vi "Query-ControlSignal.vi"(8 "error in (no error)":errorcluster, 10 "Output channel":T1, 11 "VISA resource name":refnum<visa-resource-name>) -> (0 "error out":errorcluster, 2 "Recalled Control signal / V":dbl, 3 "VISA resource name out":refnum<visa-resource-name>)   [LabVIEW 2014, in "YbTempCtrl.lvlib"]
doc: "Get the currently written control signal"
uses:
  YbTempCtrl.lvlib
  Typedefs/OutputChannelTypedef.ctl
panel:
  out "read buffer":string
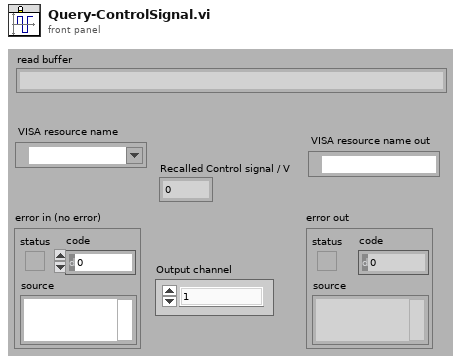
[diagram p1: front panel]
types:
  T1 = typedef "YbTempCtrl.lvlib/OutputChannelTypedef.ctl" = enum16{"1", "2", "3", "4", "BPA", "BPB"}
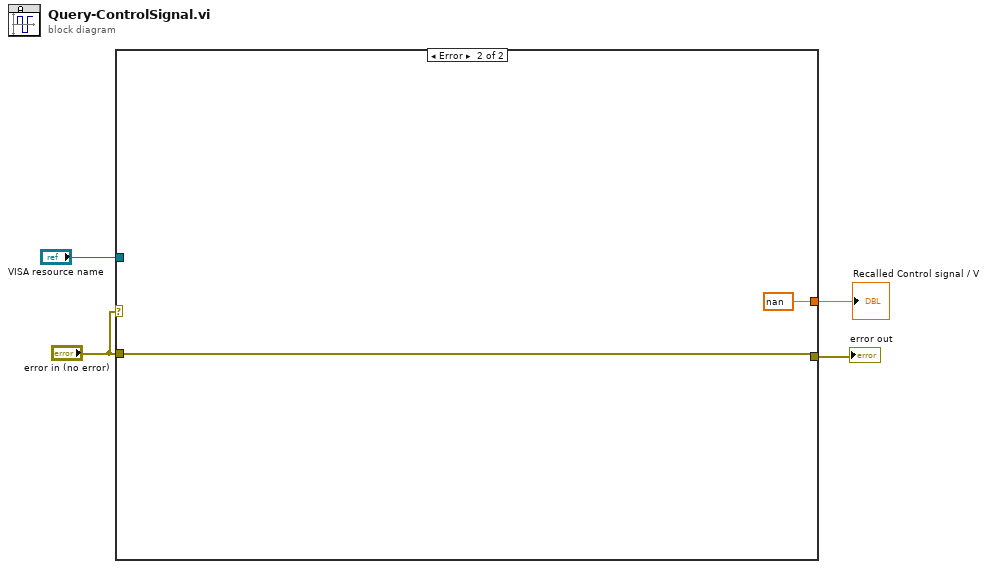
[diagram p0: block diagram]
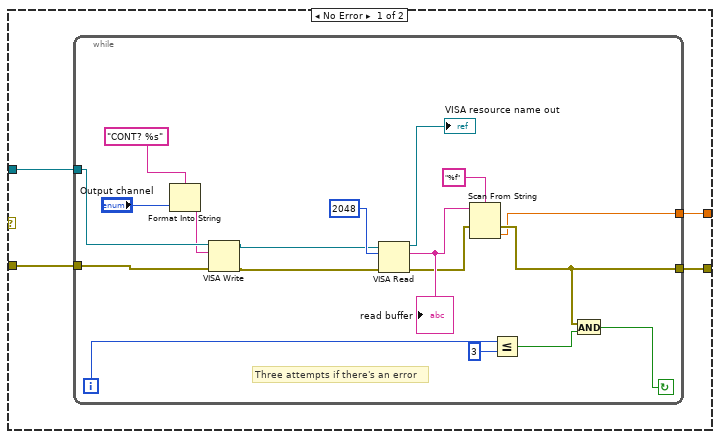
[diagram p2: hidden frame]
diagram:
  n1 = case shown="Error" "error in (no error)" {
    tunnel: "VISA resource name" -> [w8 _]
    tunnel: "error in (no error)" -> [w7 w28]
    tunnel: [w6 w28] -> w3
    tunnel: [w5 nan] -> w2
    frame No Error {
      n2 = while {
        tunnel: w8 -> [w26]
        tunnel: w7 -> [w24]
        tunnel: [w19] -> w6
        tunnel: [w10] -> w5
        i -> [w18]
        stop <- w15 continue-if-true
        # "Three attempts if there's an error"
        n3 = Format Into String(format string="CONT? %s" ("write buffer"), "Output channel") -> (resulting string=w14:string)  [unwired: 2 in, 1 out]
        n4 = VISA Write(VISA resource name=w26, write buffer=w14, error in (no error)=w24) -> (VISA resource name out=w12:refnum<visa-resource-name>, error out=w11:errorcluster)  [unwired: 1 out]
        n5 = VISA Read(VISA resource name=w12, byte count=u32 2048, error in (no error)=w11) -> (VISA resource name out=→"VISA resource name out":refnum<visa-resource-name>, read buffer=w22:string, error out=w20:errorcluster)  [unwired: 1 out]
        "read buffer" <- w22
        n6 = Scan From String(format string="%f", input string=w22, error in=w20) -> (error out=w19:errorcluster, output 1=w10:dbl)  [unwired: 2 in, 2 out]
        n7 = Less Or Equal?(x=w18, y=3) -> (x <= y?=w16:bool)
        n8 = And(x=w19, y=w16) -> (x .and. y?=w15:bool)
      }
    }
    frame Error {
    }
  }
  "error out" <- w3
  "Recalled Control signal / V" <- w2
